vi "button_main.vi"() -> ()   [LabVIEW 2023]
panel:
  out "Start_aux":bool
  in  "Start":bool
  in  "Stop Button":bool
  # "Start button launches a subvi\nThe button also stops the subvi"
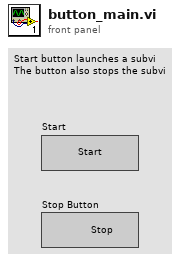
[diagram p1: front panel]
types:
  T1 = enum32{"Bad", "Idle", "Run top level", "Running"}
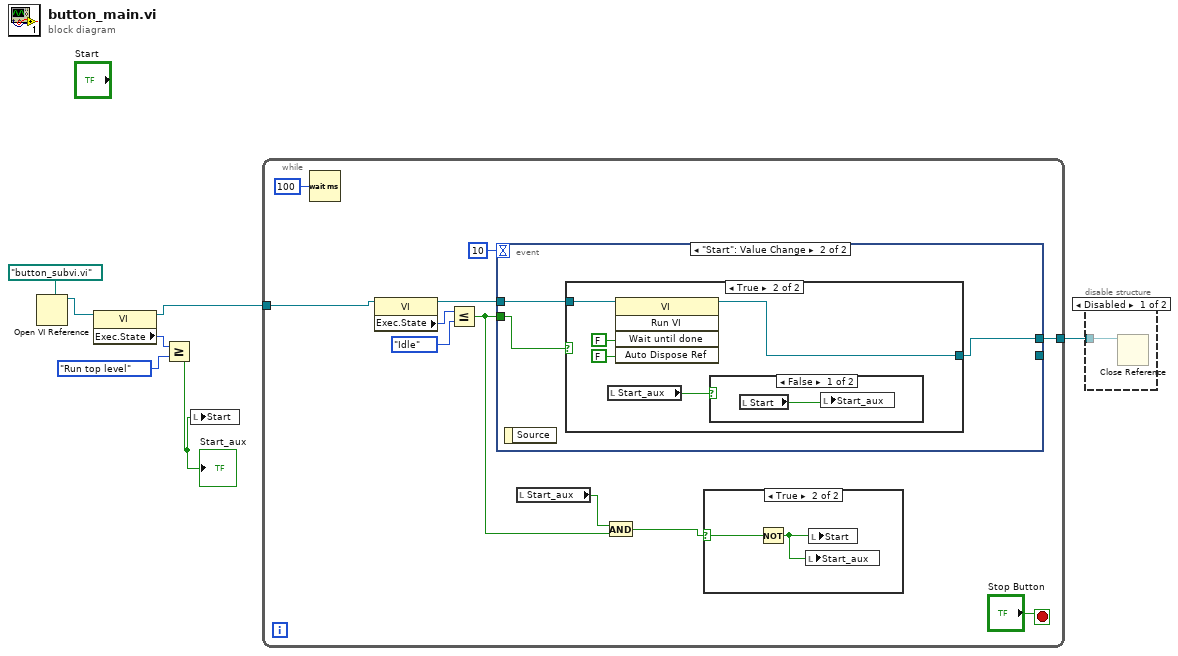
[diagram p0: block diagram]
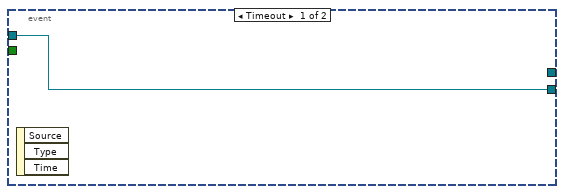
[diagram p3: hidden frame]
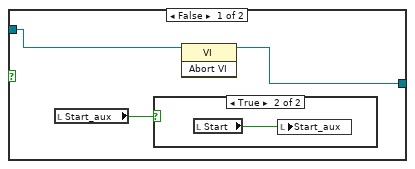
[diagram p4: hidden frame]
diagram:
  n1 = Open VI Reference(vi path=path "button_subvi.vi") -> (vi reference=w3:refnum<vi>)  [unwired: 5 in, 1 out]
  n2 = property class="VI"(reference=w3) -> (reference out=w2:refnum<vi>, "Exec.State"=w4:T1)  [unwired: 1 in, 1 out]
  n3 = Greater Or Equal?(x=w4, y=T1."Run top level" ("Execution:State")) -> (x >= y?=w1:bool)
  "Start_aux" <- w1
  n4 = local write "Start"(w1) -> ()
  n5 = while {
    tunnel: w2 -> [w9]
    tunnel: [w8] -> w6
    stop <- "Stop Button" stop-if-true
    n6 = Wait (ms)(milliseconds to wait=u32 100) -> ()  [unwired: 1 out]
    n7 = property class="VI"(reference=w9) -> (reference out=w11:refnum<vi>, "Exec.State"=w12:T1)  [unwired: 1 in, 1 out]
    n8 = Less Or Equal?(x=w12, y=T1."Idle" ("Execution:State")) -> (x <= y?=w10:bool)
    n9 = event shown="[1] \"Start\": Value Change" {
      selector: _ -> [_ _]
      dyn-events: _ -> [_ _]
      timeout: 10 -> [_ _]
      tunnel: w11 -> [w19 w21]
      tunnel: w10 -> [_ w22]
      tunnel: [w19 _] -> _
      tunnel: [_ w20] -> w8
      event Timeout {
        n10 = event-data() -> ()  [unwired: 1 in, 3 out]
      }
      event "Start": Value Change {
        n11 = event-data() -> ()  [unwired: 1 in, 1 out]
        n12 = case shown="True" w22 {
          tunnel: w21 -> [w25 w29]
          tunnel: [w24 w28] -> w20
          frame False {
            n13 = local read "Start_aux"() -> (w23:bool)
            n14 = case shown="True" w23 {
              frame False {
              }
              frame True {
                n15 = local read "Start"() -> (w26:bool)
                n16 = local write "Start_aux"(w26) -> ()
              }
            }
            n17 = invoke class="VI" method="Abort VI"(reference=w25) -> (reference out=w24:refnum<vi>)  [unwired: 2 in, 2 out]
          }
          frame True {
            n18 = local read "Start_aux"() -> (w27:bool)
            n19 = invoke class="VI" method="Run VI"(reference=w29, "Wait until done"=FALSE ("Wait Until Done"), "Auto Dispose Ref"=FALSE ("Auto Dispose Reference")) -> (reference out=w28:refnum<vi>)  [unwired: 2 in, 4 out]
            n20 = case shown="False" w27 {
              frame False {
                n21 = local read "Start"() -> (w32:bool)
                n22 = local write "Start_aux"(w32) -> ()
              }
              frame True {
              }
            }
          }
        }
      }
    }
    n23 = local read "Start_aux"() -> (w14:bool)
    n24 = And(x=w14, y=w10) -> (x .and. y?=w15:bool)
    n25 = case shown="True" w15 {
      selector: w15 -> [_ w34]
      frame False {
      }
      frame True {
        n26 = Not(x=w34) -> (.not. x?=w33:bool)
        n27 = local write "Start_aux"(w33) -> ()
        n28 = local write "Start"(w33) -> ()
      }
    }
  }
  n29 = disable-structure shown="Disabled" {
    disable-tunnel: w6 -> [w35 _]
    frame Disabled {
      n30 = Close Reference(reference=w35) -> ()  [unwired: 1 in, 1 out]
    }
    frame Enabled {
    }
  }
